vi "Move Linear Actuator.vi"(3 "error in":errorcluster, 6 "linear actuator info":T1={"distance mm"=100, "Direction"=FALSE, "speed (mm/s)"=0} {"speed (mm/s)" scale=0.0..49.0}) -> (0 "error out":errorcluster, 1 "mm/s (timed)":dbl, 2 "completed motion":bool)   [LabVIEW 2012]
uses:
  <vilib>/DAQmx/configure/timing.llb/DAQmx Timing (Implicit).vi
  <resource>/objmgr/daqmx.rc
panel:
  out "samples":i32
  out "pulse 1/2 len (ms)":dbl
  # "=17400 to go across"
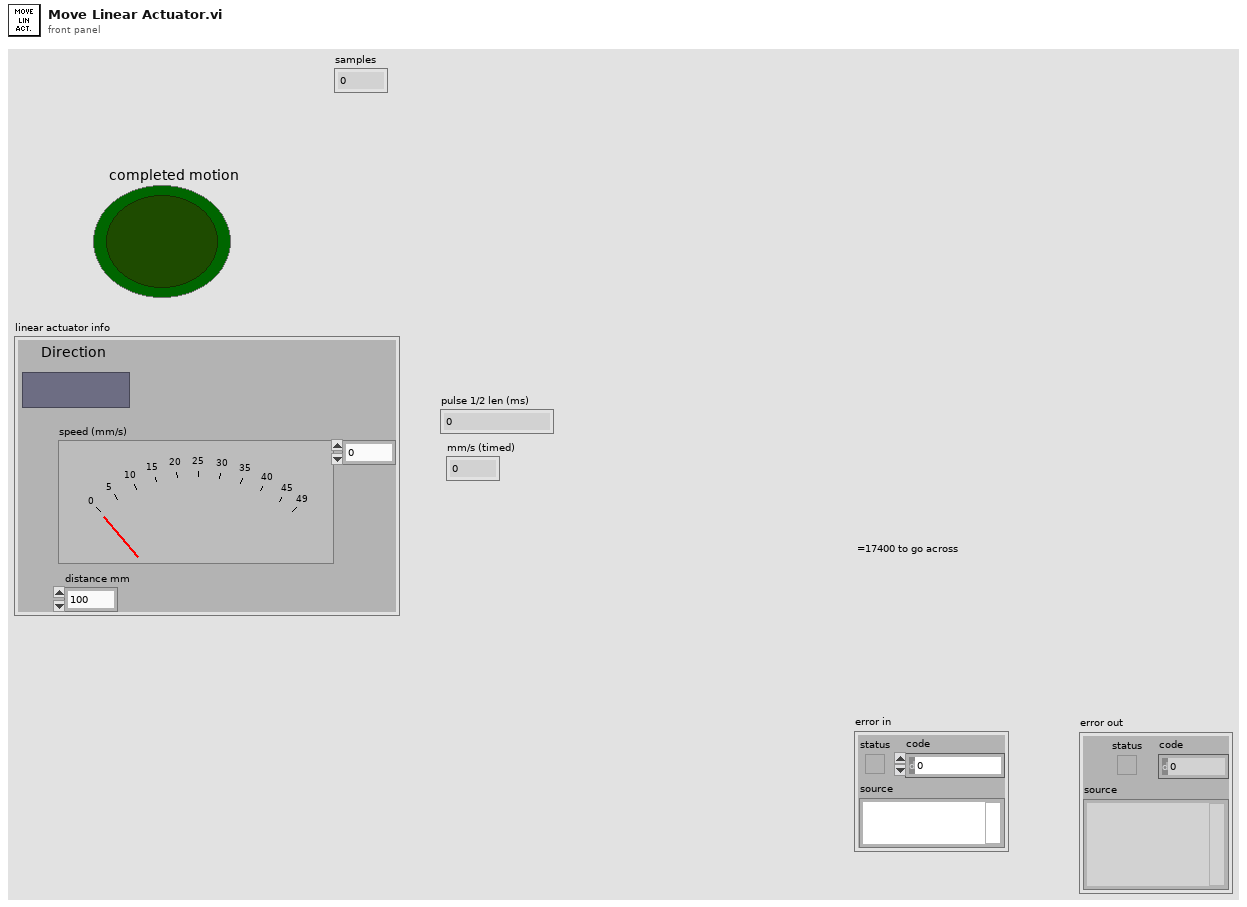
[diagram p1: front panel]
types:
  T1 = cluster{"distance mm":i32, "Direction":bool, "speed (mm/s)":i32}
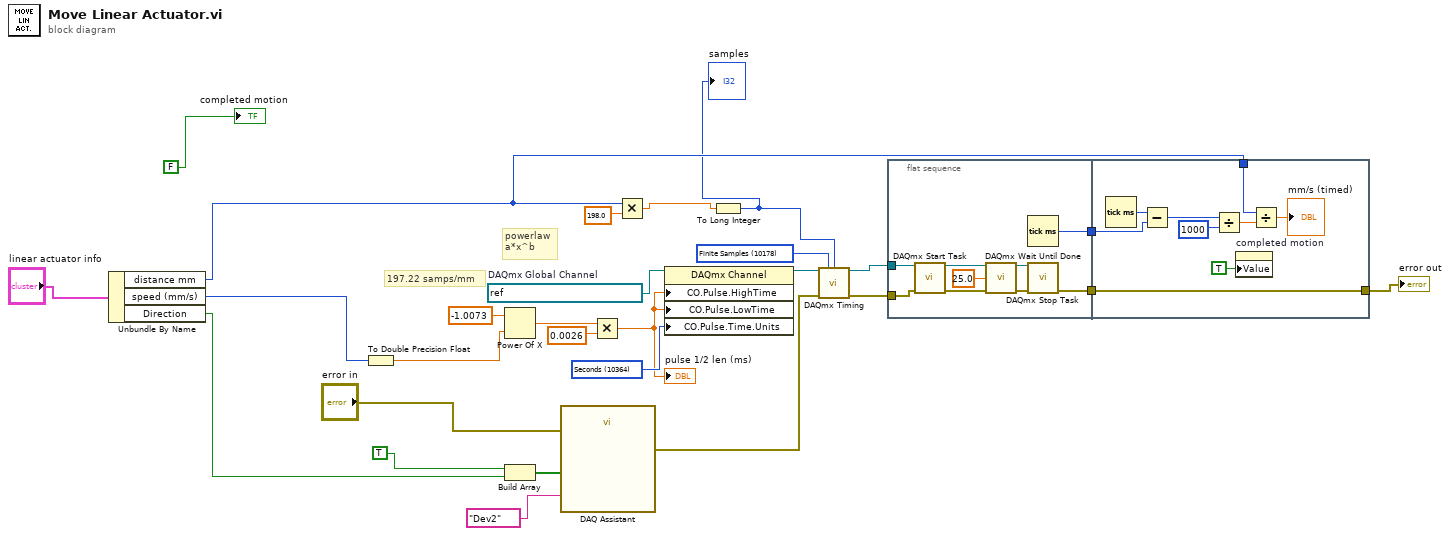
[diagram p0: block diagram]
diagram:
  w24 = 10364 items=["Seconds"=10364] ("CO.Pulse.Time.Units")
  w21 = 10178 items=["Finite Samples"=10178, "Continuous Samples"=10123, "Hardware Timed Single Point"=12522] ("sample mode")
  w20 = refnum<k21> "MyPulseOutputChannel"  # DAQmx Global Channel
  # "powerlaw\na*x^b"
  # "197.22 samps/mm"
  n1 = Unbundle By Name("linear actuator info") -> ("distance mm"=w4:i32, "speed (mm/s)"=w5:i32, "Direction"=w6:bool)
  n2 = To Double Precision Float(number=w5) -> (double precision float=w3:dbl)
  n3 = Power Of X(1:w3, 2:-1.0073) -> (0:w16:dbl)
  n4 = Build Array(TRUE ("element"), w6) -> (w19:bool[])
  n5 = call "DAQ Assistant"("data"=w19, "error in"="error in", "device name"=tag "Dev2") -> ("error out"=w10:errorcluster)  [unwired: 15 in, 1 out]
  n6 = Multiply(x=w16, y=0.0026) -> (x*y=w14:dbl)
  "pulse 1/2 len (ms)" <- w14
  n7 = Multiply(x=w4, y=198.0) -> (x*y=w2:dbl)
  n8 = property class="DAQmx Channel"(reference=w20, "CO.Pulse.HighTime"=w14, "CO.Pulse.LowTime"=w14, "CO.Pulse.Time.Units"=w24) -> (reference out=w23:refnum<k21>)  [unwired: 1 in, 1 out]
  n9 = To Long Integer(number=w2) -> (32bit integer=w1:i32)
  "samples" <- w1
  n10 = call-poly <vilib>:"DAQmx Timing.vi"("task/channels in"=w23, "sample mode"=w21, "samples per channel"=w1, "error in"=w10) -> ("task out"=w22:refnum<k21>, "error out"=w11:errorcluster)  [unwired: 10 in]
  n11 = flat-sequence {
    tunnel: w22 -> [w34]
    tunnel: [w30] -> w27
    tunnel: [w29] -> w26
    tunnel: w11 -> [w28]
    tunnel: w27 -> [w45]
    tunnel: w4 -> [w41]
    tunnel: w26 -> [w38]
    tunnel: [w38] -> w12
    frame #0 {
      n12 = call <vilib>:"DAQmx Start Task.vi"("task/channels in"=w34, "error in"=w28) -> ("task out"=w35:refnum<k21>, "error out"=w32:errorcluster)  [unwired: 12 in]
      n13 = call <vilib>:"DAQmx Wait Until Done.vi"("task/channels in"=w35, "timeout (sec)"=25.0, "error in"=w32) -> ("task out"=w33:refnum<k21>, "error out"=w31:errorcluster)  [unwired: 11 in]
      n14 = Tick Count (ms)() -> (millisecond timer value=w30:u32)
      n15 = call <vilib>:"DAQmx Stop Task.vi"("task/channels in"=w33, "error in"=w31) -> ("error out"=w29:errorcluster)  [unwired: 12 in, 1 out]
    }
    frame #1 {
      n16 = Tick Count (ms)() -> (millisecond timer value=w44:u32)
      n17 = Subtract(x=w44, y=w45) -> (x-y=w43:u32)
      n18 = Divide(x=w43, y=u32 1000) -> (x/y=w40:dbl)
      n19 = property on="completed motion" class="Bool (strict)"("Value"=TRUE ("completed motion")) -> ()  [unwired: 2 in, 2 out]
      n20 = Divide(x=w41, y=w40) -> (x/y=→"mm/s (timed)":dbl)
    }
  }
  "error out" <- w12
  "completed motion" <- FALSE
